vi "Add From Spreadsheet.vi"(7 "file path (use dialog)":path, 8 "error in (no error)":errorcluster, 11 "Item Ref":T1 format="%.0x") -> (0 "error out":errorcluster)   [LabVIEW 2017, in "GE_RM_System Explorer.lvlib"]
uses:
  GE_RM_System Explorer.lvlib
  <vilib>/NI Veristand/Custom Device API/Custom Device Item Ref.ctl
  <vilib>/NI Veristand/Custom Device API/Custom Device Channel.ctl
  <vilib>/NI Veristand/Custom Device API/Custom Device Channel Type.ctl
  Shared/Data Channel Type.ctl
  <vilib>/NI Veristand/Custom Device API/Set Item Property (U32).vi
  <vilib>/NI Veristand/Custom Device API/Set Item Property (U16).vi
  Shared/Global.vi
  Shared/GE_RM_Shared.lvlib
  <vilib>/NI VeriStand/Custom Device API/Custom Device API.lvlib
panel:
  out "array w/ subset deleted":string[][](array[string])
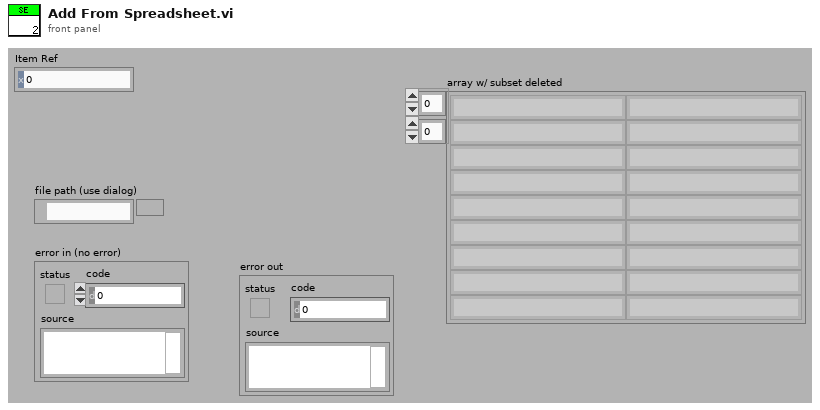
[diagram p1: front panel]
types:
  T1 = typedef "Custom Device API.lvlib/Custom Device Item Ref.ctl" = u64
  T2 = typedef "Custom Device API.lvlib/Custom Device Channel.ctl" = cluster{"Type":T3, "Units":string, "Default Value":dbl, "Faultable":bool, "Scalable":bool}
  T3 = typedef "Custom Device API.lvlib/Custom Device Channel Type.ctl" = enum16{"Input", "Output"}
  T4 = typedef "GE_RM_System Explorer.lvlib/Data Channel Type.ctl" = enum16{"Read", "Write"}
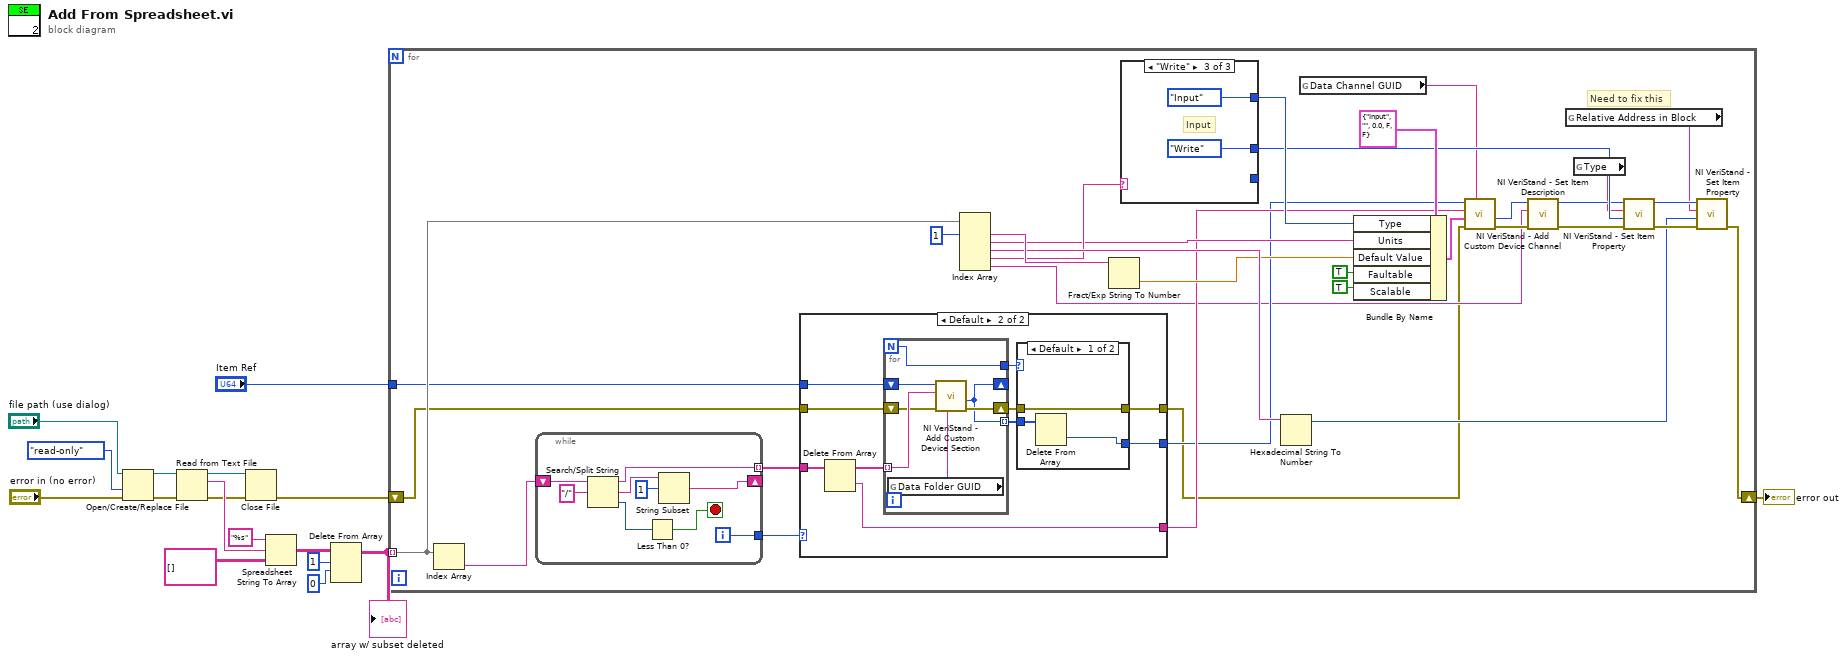
[diagram p0: block diagram]
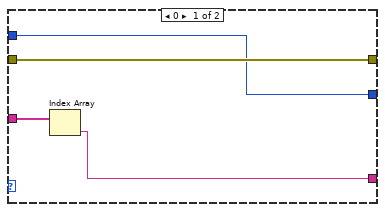
[diagram p2: hidden frame]
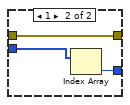
[diagram p3: hidden frame]
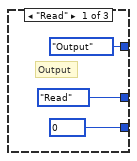
[diagram p4: hidden frame]
diagram:
  n1 = Open/Create/Replace File(file path (use dialog)="file path (use dialog)", error in="error in (no error)", access (0:read/write)=enum16{"read/write", "read-only", "write-only"}."read-only") -> (refnum out=w7:refnum<file>, error out=w6:errorcluster)  [unwired: 3 in, 1 out]
  n2 = Read from Text File(file (use dialog)=w7, error in=w6) -> (refnum out=w8:refnum<file>, text=w11:string, error out=w9:errorcluster)  [unwired: 2 in, 1 out]
  n3 = Close File(refnum=w8, error in=w9) -> (error out=w17:errorcluster)  [unwired: 1 out]
  n4 = Spreadsheet String To Array(format string="%s", spreadsheet string=w11, array type (2D Dbl)=string[][] []) -> (array=w13:string[][])  [unwired: 1 in]
  n5 = Delete From Array(array=w13, length=1, index (row)=0) -> (array with subset deleted=w16:string[][])  [unwired: 1 in, 1 out]
  "array w/ subset deleted" <- w16
  n6 = for {
    tunnel: w16 -> [w50] mode=indexing
    shift-right: [w18] -> w1
    shift-left: w17 -> [w23]
    tunnel: "Item Ref" -> [w30]
    # "Need to fix this"
    n7 = Index Array(array=w50) -> (element=w32:string)  [unwired: 1 in]
    n8 = while {
      tunnel: [w82] -> w33 mode=indexing
      shift-right: [w80] -> _
      shift-left: w32 -> [w86]
      tunnel: [w78] -> w34
      i -> [w78]
      stop <- w83 stop-if-true
      n9 = Search/Split String(string=w86, search string/char (-)="/") -> (substring before match=w82:string, match + rest of string=w81:string, offset of match=w84:i32)  [unwired: 1 in]
      n10 = Less Than 0?(x=w84) -> (x < 0?=w83:bool)
      n11 = String Subset(string=w81, offset (0)=1) -> (substring=w80:string)  [unwired: 1 in]
    }
    n12 = case shown="Default" w34 {
      tunnel: [w54 w58] -> w19
      tunnel: w23 -> [w54 w63]
      tunnel: w33 -> [w53 w64]
      tunnel: w30 -> [w51 w56]
      tunnel: [w52 w57] -> w31
      tunnel: [w51 w55] -> w29
      frame 0 {
        n13 = Index Array(array=w53) -> (element=w52:string)  [unwired: 1 in]
      }
      frame Default {
        n14 = Delete From Array(array=w64) -> (deleted portion=w57:string, array with subset deleted=w62:string[])  [unwired: 2 in]
        n15 = for {
          N -> [w77]
          shift-right: [w73] -> w59
          shift-left: w63 -> [w74]
          shift-right: [w71] -> _
          shift-left: w56 -> [w72]
          tunnel: w62 -> [w76] mode=indexing
          tunnel: [w71] -> w60 mode=indexing
          tunnel: [w77] -> w61
          n16 = global read "Global.vi" "Data Folder GUID"() -> (w75:string)
          n17 = call <vilib>:"NI VeriStand - Add Custom Device Section.vi"("GUID (Default Section)"=w75, "error in (no error)"=w74, "Section Name"=w76, "Parent Ref in"=w72) -> ("error out"=w73:errorcluster, "Section Ptr"=w71:T1)  [unwired: 4 in, 2 out]
        }
        n18 = case shown="Default" w61 {
          tunnel: w60 -> [w67 w70]
          tunnel: [w66 w69] -> w55
          tunnel: w59 -> [w65 w68]
          tunnel: [w65 w68] -> w58
          frame Default {
            n19 = Delete From Array(array=w67) -> (deleted portion=w66:T1)  [unwired: 2 in, 1 out]
          }
          frame 1 {
            n20 = Index Array(array=w70) -> (element=w69:T1)  [unwired: 1 in]
          }
        }
      }
    }
    n21 = Index Array(array=w50, index #1=1 ("index")) -> (element #1=w48:string, element #2=w43:string, element #3=w47:string, element #4=w46:string, element #5=w25:string)  [unwired: 4 in]
    n22 = Fract/Exp String To Number(string=w48) -> (number=w42:dbl)  [unwired: 3 in, 1 out]
    n23 = case shown="\"Write\"" w46 {
      tunnel: [Data_Channel_Type."Read" ("Type") _ Data_Channel_Type."Write" ("Type")] -> w38
      tunnel: [u32 0 ("BitFields") _ _] -> _
      tunnel: [Custom_Device_Channel_Type."Output" ("Type") _ Custom_Device_Channel_Type."Input" ("Type")] -> w39
      frame "Read" {
        # "Output"
      }
      frame Default {
      }
      frame "Write" {
        # "Input"
      }
    }
    n24 = Hexadecimal String To Number(string=w47) -> (number=w35:u32)  [unwired: 2 in, 1 out]
    n25 = global read "Global.vi" "Data Channel GUID"() -> (w20:string)
    n26 = Bundle By Name(cluster=T2 {"Type"=enum."Input", "Units"="", "Default Value"=0.0, "Faultable"=FALSE, "Scalable"=FALSE} ("Channel"), "Type"=w39, "Units"=w43, "Default Value"=w42, "Faultable"=TRUE, "Scalable"=TRUE) -> (w44:T2)
    n27 = call <vilib>:"NI VeriStand - Add Custom Device Channel.vi"("GUID (Default Channel)"=w20, "error in (no error)"=w19, "Channel"=w44, "Channel Name"=w31, "Parent Ref in"=w29) -> ("error out"=w28:errorcluster, "Channel Ref"=w24:T1)  [unwired: 3 in, 2 out]
    n28 = call <vilib>:"NI VeriStand - Set Item Description.vi"("error in (no error)"=w28, "Description"=w25, "Item Ref in"=w24) -> ("error out"=w27:errorcluster, "Item Ref out"=w26:T1)  [unwired: 6 in, 1 out]
    n29 = global read "Global.vi" "Relative Address in Block"() -> (w22:string)
    n30 = global read "Global.vi" "Type"() -> (w21:string)
    n31 = call-poly <vilib>:"NI VeriStand - Set Item Property.vi"("error in (no error)"=w27, "Value"=w38, "Property Name"=w21, "Item Ref in"=w26) -> ("error out"=w36:errorcluster, "Item Ref out"=w37:T1)  [unwired: 5 in, 1 out]
    n32 = call-poly <vilib>:"NI VeriStand - Set Item Property.vi"("error in (no error)"=w36, "Value"=w35, "Property Name"=w22, "Item Ref in"=w37) -> ("error out"=w18:errorcluster)  [unwired: 5 in, 2 out]
  }
  "error out" <- w1
